vi "communicateMLCStart.vi"(8 "error in (no error)":errorcluster) -> (0 "error out":errorcluster, 3 "message out":T1=enum."end")   [LabVIEW 2017, in "communicateMLC.lvlib"]
uses:
  communicateMLC.lvlib
  TypeDefs/LoopStates.ctl
  programControl/StartUEFGV/TypeDefs/UEFGVcontrol.ctl
  programControl/programControl.lvlib
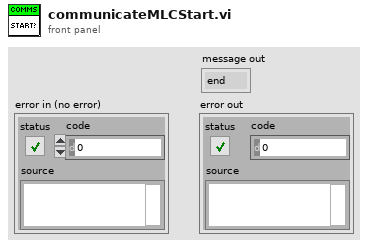
[diagram p1: front panel]
types:
  T1 = typedef "LoopStates.ctl" = enum16{"start", "wait", "run", "end"}
  T2 = typedef "UEFGVcontrol.ctl" = enum16{"Create", "Get", "Destroy"}
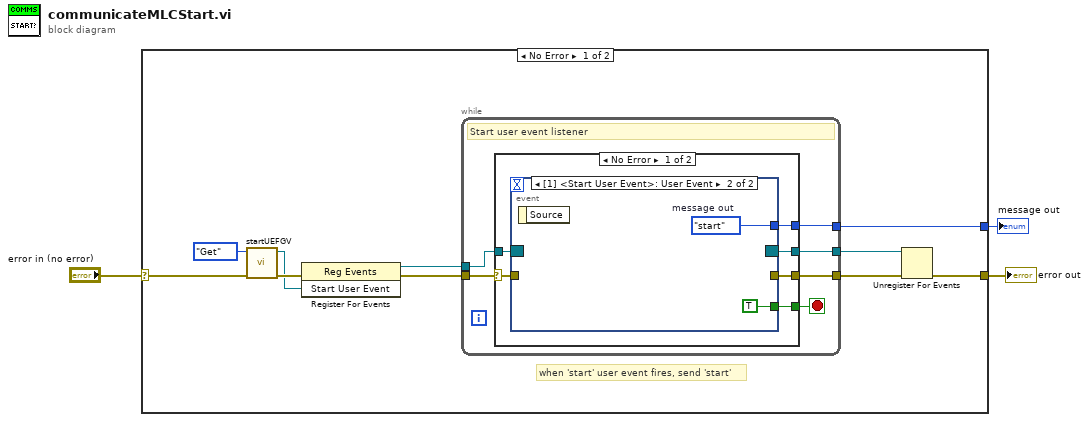
[diagram p0: block diagram]
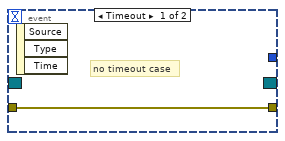
[diagram p2: hidden frame]
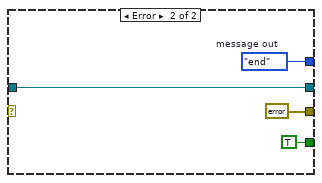
[diagram p3: hidden frame]
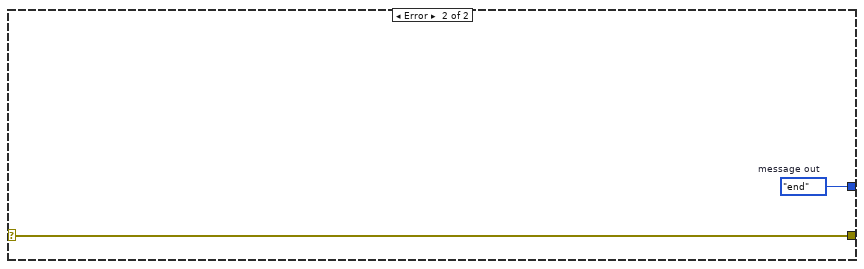
[diagram p4: hidden frame]
diagram:
  n1 = case shown="No Error" "error in (no error)" {
    selector: "error in (no error)" -> [w13 w34]
    tunnel: [w6 w34] -> w3
    tunnel: [w4 w33] -> w1
    frame No Error {
      # "when 'start' user event fires, send 'start'"
      n2 = call "startUEFGV.vi"("error in (no error)"=w13, "Enum"=UEFGVcontrol."Get") -> ("error out"=w11:errorcluster, "Start User Event"=w10:refnum<user-event>)  [unwired: 8 in]
      n3 = register-events(error in=w11, w10) -> (reference out=w8:refnum<event-registration>, error out=w9:errorcluster)  [unwired: 1 in]
      n4 = while {
        tunnel: w8 -> [w19]
        tunnel: [w18] -> w5
        tunnel: w9 -> [w16]
        tunnel: [w15] -> w7
        tunnel: [w14] -> w4
        stop <- w17 stop-if-true
        # "Start user event listener"
        n5 = case shown="No Error" w16 {
          selector: w16 -> [w22 _]
          tunnel: w19 -> [w25 w31]
          tunnel: [w24 w31] -> w18
          tunnel: [w23 TRUE] -> w17
          tunnel: [w21 errorcluster {"status"=FALSE, "code"=0, "source"=""} ("error out")] -> w15
          tunnel: [w20 w29] -> w14
          frame No Error {
            n6 = event shown="[1] <Start User Event>: User Event" {
              selector: w25 -> [_ _]
              dyn-events: [_ _] -> w24
              timeout: _ -> [_ _]
              tunnel: w22 -> [w26 _]
              tunnel: [w26 _] -> w21
              tunnel: [_ TRUE] -> w23
              tunnel: [_ w27] -> w20
              event Timeout {
                # "no timeout case"
                n7 = event-data() -> ()  [unwired: 1 in, 3 out]
              }
              event User Event {
                w27 = LoopStates."start"  # message out
                n8 = event-data() -> ()  [unwired: 1 in, 1 out]
              }
            }
          }
          frame Error {
            w29 = LoopStates."end"  # message out
          }
        }
      }
      n9 = Unregister For Events(event registration refnum=w5, error in=w7) -> (error out=w6:errorcluster)
    }
    frame Error {
      w33 = LoopStates."end"  # message out
    }
  }
  "error out" <- w3
  "message out" <- w1
